vi "Get Result.vi"(4 "Controller name":string, 6 "Last request":bool, 8 "error in (no error)":errorcluster, 11 "Instrument Recorder in":refnum<class "Pulse Recorder Actor.lvclass">) -> (0 "error out":errorcluster, 2 "Result":refnum<class "Acquired Result.lvclass">, 3 "Instrument Recorder out":refnum<class "Pulse Recorder Actor.lvclass">)   [LabVIEW 2021, in "Pulse Recorder Actor.lvclass"]
uses:
  Pulse Recorder Actor.lvclass
  Pulse Recorder Actor.lvclass/Pulse Recorder Actor.ctl
  Instrument Actor/Instrument Actor.lvclass
  NHMFL_Core/Libraries/Instruments/Results/Acquired Result/Acquired Result.lvclass
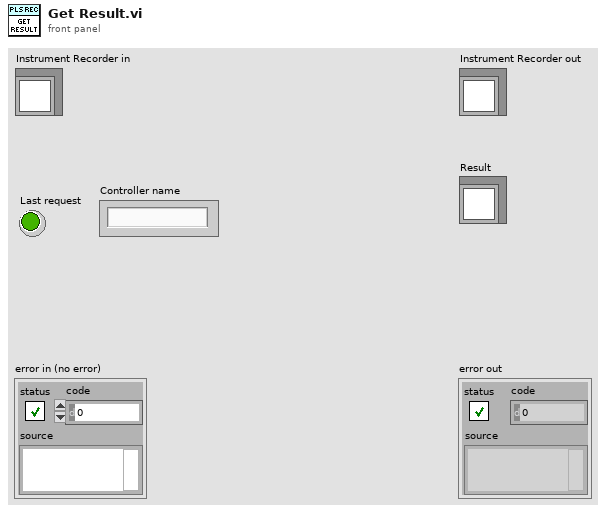
[diagram p1: front panel]
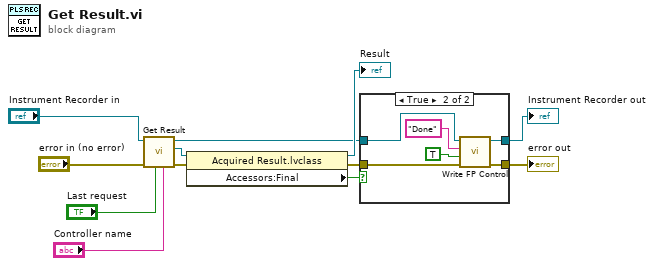
[diagram p0: block diagram]
diagram:
  n1 = call-parent "Get Result.vi"("Controller name"="Controller name", "Last request"="Last request", "error in (no error)"="error in (no error)", "Instrument Recorder in"="Instrument Recorder in") -> ("error out"=w12:errorcluster, "Result"=w8:refnum<class "Acquired Result.lvclass">, "Instrument Recorder out"=w2:refnum<class "Pulse Recorder Actor.lvclass">)  [unwired: 5 in]
  n2 = property class="Acquired Result.lvclass"(reference=w8, error in=w12) -> (reference out=→"Result":refnum<class "Acquired Result.lvclass">, error out=w5:errorcluster, "Accessors:Final"=w6:bool)
  n3 = case shown="True" w6 {
    tunnel: w5 -> [w14 w18]
    tunnel: [w14 w17] -> w4
    tunnel: [w13 w16] -> w3
    tunnel: w2 -> [w13 w15]
    frame False {
    }
    frame True {
      n4 = call-dynamic "Write FP Control.vi"("error in (no error)"=w18, "Control Value"=TRUE, "Control Name"="Done", "Measure Object in"=w15) -> ("error out"=w17:errorcluster, "Measure Object out"=w16:refnum<class "Pulse Recorder Actor.lvclass">)  [unwired: 6 in]
    }
  }
  "error out" <- w4
  "Instrument Recorder out" <- w3
